vi "WRITE File.vi"(0 "reference in":refnum<class "RPC.lvclass">, 5 "error in (no error)":errorcluster, 7 "MegaDAC RPC File (*.rsp)":path) -> (14 "reference out":refnum<class "RPC.lvclass">, 19 "error out":errorcluster)   [LabVIEW 2020, in "RPC.lvclass"]
uses:
  RPC.lvclass
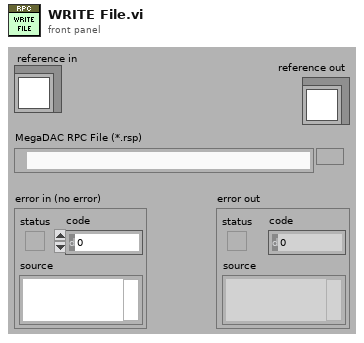
[diagram p1: front panel]
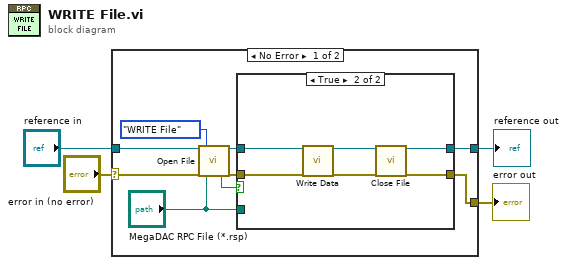
[diagram p0: block diagram]
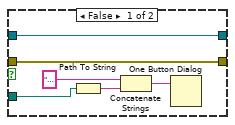
[diagram p2: hidden frame]
diagram:
  n1 = case shown="No Error" "error in (no error)" {
    selector: "error in (no error)" -> [w12 w27]
    tunnel: [w8 w27] -> w3
    tunnel: [w9 w26] -> w1
    tunnel: "reference in" -> [w13 w26]
    frame No Error {
      n2 = call "Open File.vi"("reference in"=w13, "error in (no error)"=w12, "IO Type"=enum16{"READ File", "WRITE File"}."WRITE File", "MegaDAC RPC File (*.rsp)"="MegaDAC RPC File (*.rsp)") -> ("file or folder exists?"=w7:bool, "reference out"=w10:refnum<class "RPC.lvclass">, "error out"=w11:errorcluster)  [unwired: 13 in]
      n3 = case shown="True" w7 {
        tunnel: w11 -> [w18 w22]
        tunnel: w10 -> [w19 w23]
        tunnel: [w19 w25] -> w9
        tunnel: [w18 w24] -> w8
        tunnel: "MegaDAC RPC File (*.rsp)" -> [w14 _]
        frame False {
          n4 = Path To String(path=w14) -> (string=w15:string)
          n5 = Concatenate Strings("Warning, the MegaDAC File (*.rsp) cannot be saved?\n" ("message"), w15) -> (w16:string)
          n6 = One Button Dialog(message=w16) -> ()  [unwired: 1 in, 1 out]
        }
        frame True {
          n7 = call "Write Data.vi"("reference in"=w23, "error in (no error)"=w22) -> ("reference out"=w20:refnum<class "RPC.lvclass">, "error out"=w21:errorcluster)  [unwired: 16 in]
          n8 = call "Close File.vi"("reference in"=w20, "error in (no error)"=w21) -> ("reference out"=w25:refnum<class "RPC.lvclass">, "error out"=w24:errorcluster)  [unwired: 16 in]
        }
      }
    }
    frame Error {
    }
  }
  "error out" <- w3
  "reference out" <- w1
